vi "Archery_Hint.vi"() -> ()   [LabVIEW 2014]
panel:
  in  "OK":bool
  # "How to Play"
  # "1. Aim your mouse at the target, and press left mouse\n    button once to shoot an arrow.\n\n2. The arrow will be affected by gravity and wind, so\n    you need to predict how much displacement to\n    compensate.\n\n3. The target will keep moving until the arrow achieve,\n    and the flying time is proportional to the distance."
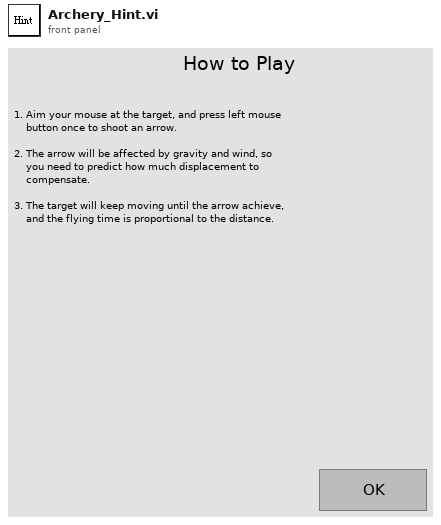
[diagram p1: front panel]
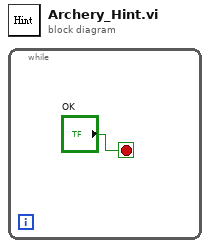
[diagram p0: block diagram]
diagram:
  n1 = while {
    stop <- "OK" stop-if-true
  }
